vi "field_to_current_convert_planar.vi"(1 "Field, Oe":dbl) -> (0 "Current, A":dbl)   [LabVIEW 2017]
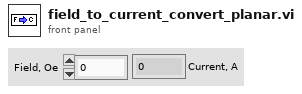
[diagram p1: front panel]
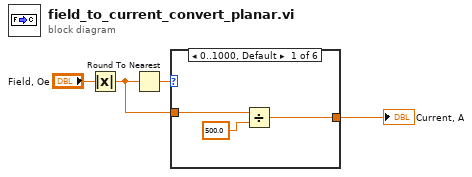
[diagram p0: block diagram]
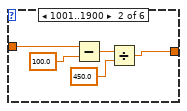
[diagram p2: hidden frame]
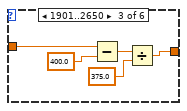
[diagram p3: hidden frame]
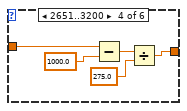
[diagram p4: hidden frame]
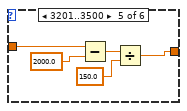
[diagram p5: hidden frame]
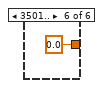
[diagram p6: hidden frame]
diagram:
  n1 = Absolute Value(x="Field, Oe") -> (abs(x)=w2:dbl)
  n2 = Round To Nearest(number=w2) -> (nearest integer value=w3:dbl)
  n3 = case shown="0..1000, Default" w3 {
    tunnel: w2 -> [w7 w12 w14 w19 w24 _]
    tunnel: [w5 w8 w13 w18 w23 0.0] -> w1
    frame 0..1000, Default {
      n4 = Divide(x=w7, y=500.0) -> (x/y=w5:dbl)
    }
    frame 1001..1900 {
      n5 = Subtract(x=w12, y=100.0) -> (x-y=w10:dbl)
      n6 = Divide(x=w10, y=450.0) -> (x/y=w8:dbl)
    }
    frame 1901..2650 {
      n7 = Subtract(x=w14, y=400.0) -> (x-y=w16:dbl)
      n8 = Divide(x=w16, y=375.0) -> (x/y=w13:dbl)
    }
    frame 2651..3200 {
      n9 = Subtract(x=w19, y=1000.0) -> (x-y=w21:dbl)
      n10 = Divide(x=w21, y=275.0) -> (x/y=w18:dbl)
    }
    frame 3201..3500 {
      n11 = Subtract(x=w24, y=2000.0) -> (x-y=w26:dbl)
      n12 = Divide(x=w26, y=150.0) -> (x/y=w23:dbl)
    }
    frame 3501.. {
    }
  }
  "Current, A" <- w1
